vi "Data Processing.vi"(7 "Start Time Stamp":timestamp, 8 "error in":errorcluster, 9 "Control Data Notifier":refnum<notifier>, 10 "Unprocessed Data":refnum<queue>, 11 "Calibration Configuration":T2) -> (0 "error out":errorcluster, 2 "Data":T1, 3 "Data w Time":T1)   [LabVIEW 2024]
uses:
  support/Control/Waveform Data Constant.ctl
  Configuration/Calibration Configuration.ctl
  support/Control/Data Constant.ctl
  support/Control/Control Data Constant.ctl
  <vilib>/Analysis/baseanly.llb/Mean (DBL).vi
  <vilib>/Waveform/DTblOps.llb/DTbl Digital to Boolean Array.vi
  <vilib>/Analysis/NI_AALBase.lvlib
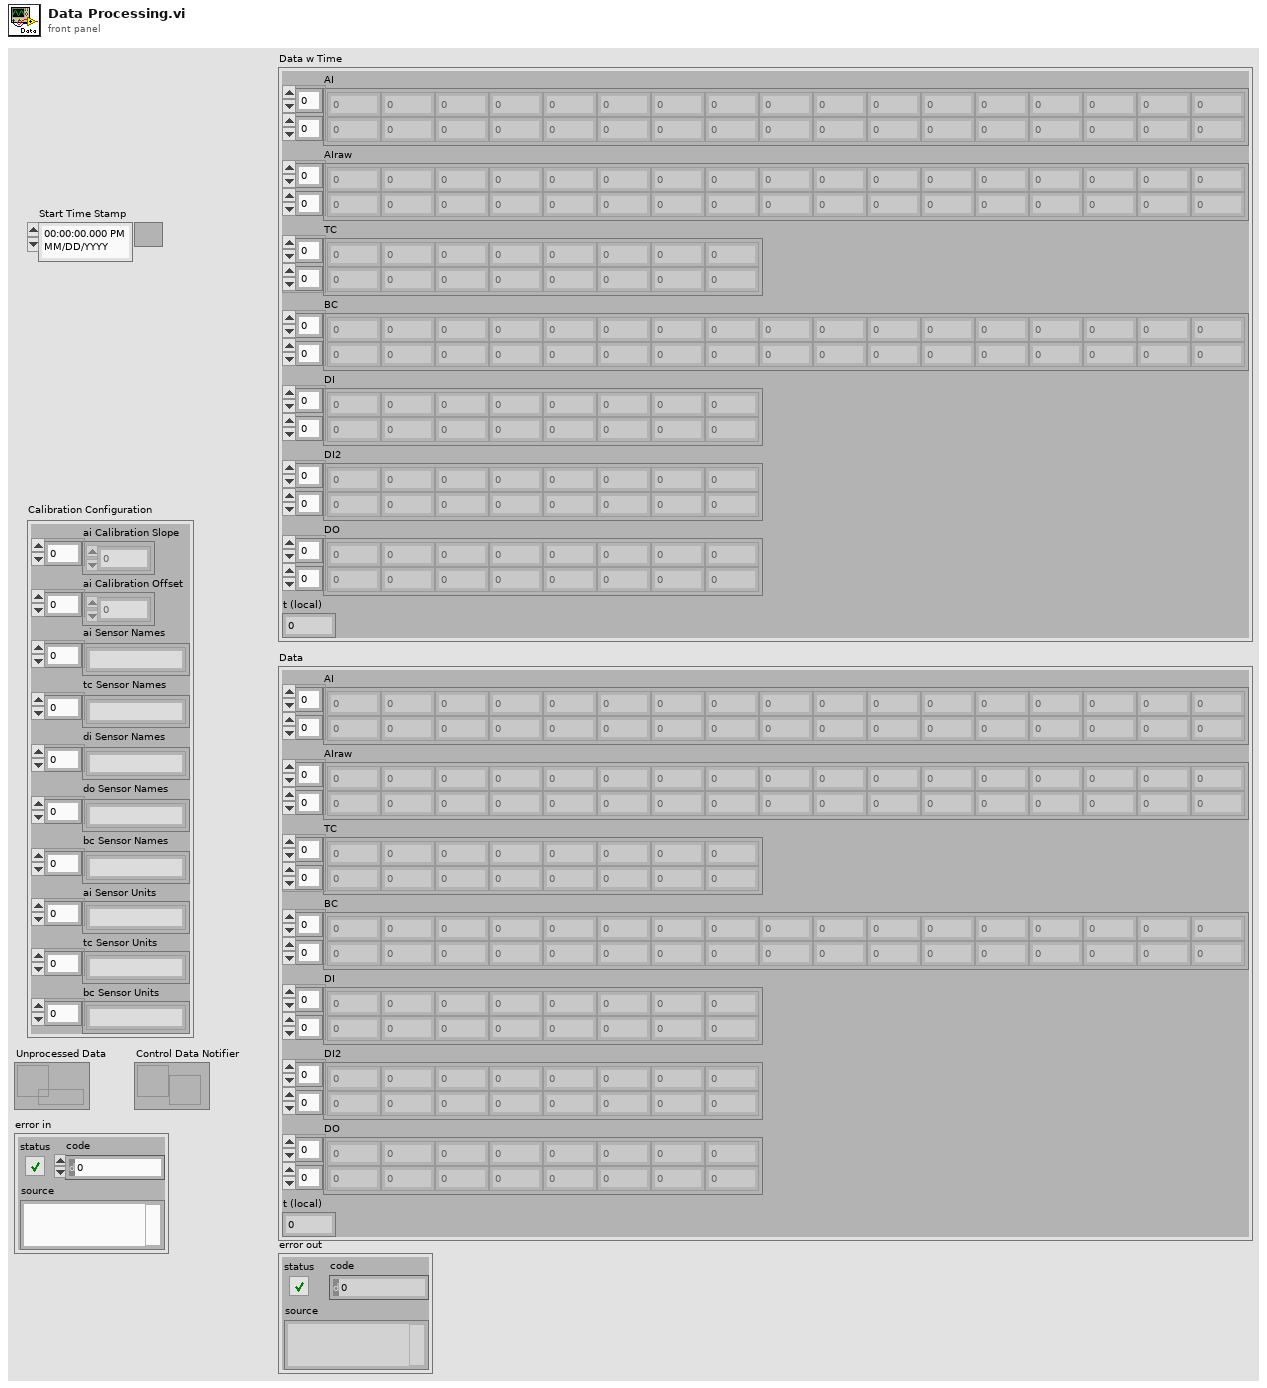
[diagram p1: front panel]
types:
  T1 = typedef "Data Constant.ctl" = cluster{"AI":dbl[][], "AIraw":dbl[][], "TC":dbl[][], "BC":dbl[][], "DI":dbl[][], "DI2":dbl[][], "DO":dbl[][], "t (local)":dbl}
  T2 = typedef "Calibration Configuration.ctl" = cluster{"ai Calibration Slope":dbl[], "ai Calibration Offset":dbl[], "ai Sensor Names ":string[], "tc Sensor Names":string[], "di Sensor Names":string[], "do Sensor Names":string[], "bc Sensor Names":string[], "ai Sensor Units":string[], "tc Sensor Units":string[], "bc Sensor Units":string[]}
  T3 = typedef "Waveform Data Constant.ctl" = cluster{"AI":waveform(dbl)[], "TC":waveform(dbl)[], "BC":waveform(dbl)[], "DI":digitalwaveform[], "DI2":digitalwaveform[]}
  T4 = typedef "Control Data Constant.ctl" = cluster{"Time (utc)":ext, "Data Out":cluster{"DO":bool[], "Module Number":string}[]}
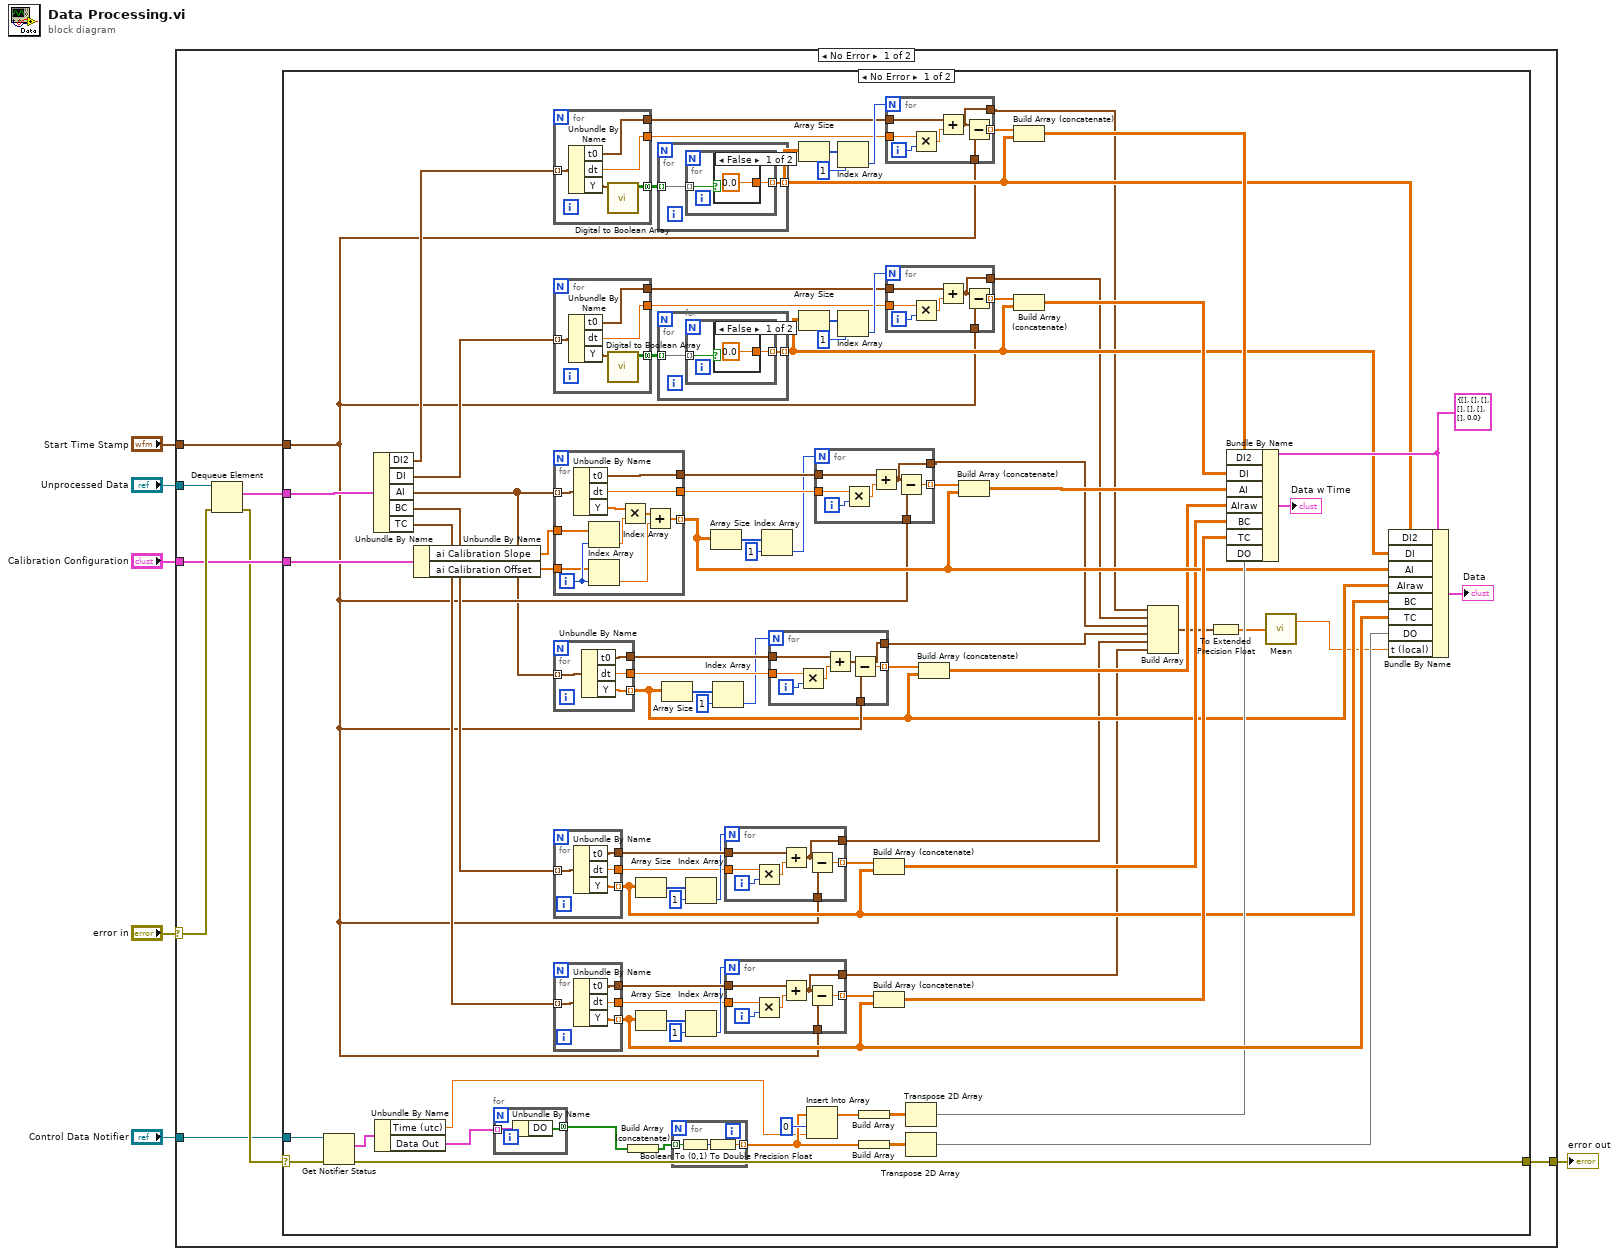
[diagram p0: block diagram]
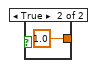
[diagram p2: hidden frame]
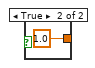
[diagram p3: hidden frame]
diagram:
  n1 = case shown="No Error" "error in" {
    selector: "error in" -> [w12 w194]
    tunnel: "Unprocessed Data" -> [w13 _]
    tunnel: [w9 w194] -> w4
    tunnel: "Calibration Configuration" -> [w11 _]
    tunnel: "Start Time Stamp" -> [w10 _]
    tunnel: "Control Data Notifier" -> [w7 _]
    frame No Error {
      n2 = Dequeue Element(queue=w13, error in (no error)=w12) -> (element=w14:T3, error out=w8:errorcluster)  [unwired: 1 in, 2 out]
      n3 = case shown="No Error" w8 {
        selector: w8 -> [w61 _]
        tunnel: w14 -> [w101 _]
        tunnel: w11 -> [w92 _]
        tunnel: w10 -> [w30 _]
        tunnel: [w60 _] -> w9
        tunnel: w7 -> [w64 _]
        frame No Error {
          w62 = T1 {"AI"=[], "AIraw"=[], "TC"=[], "BC"=[], "DI"=[], "DI2"=[], "DO"=[], "t (local)"=0.0} ("Data")
          n4 = Get Notifier Status(notifier=w64, error in (no error)=w61) -> (current notification=w42:T4, error out=w60:errorcluster)  [unwired: 3 out]
          n5 = Unbundle By Name(w101) -> ("DI2"=w52:digitalwaveform[], "DI"=w84:digitalwaveform[], "AI"=w29:waveform(dbl)[], "BC"=w80:waveform(dbl)[], "TC"=w95:waveform(dbl)[])
          n6 = Unbundle By Name(w42) -> ("Time (utc)"=w17:ext, "Data Out"=w16:cluster{"DO":bool[], "Module Number":string}[])
          n7 = Unbundle By Name(w92) -> ("ai Calibration Slope"=w91:dbl[], "ai Calibration Offset"=w90:dbl[])
          n8 = for {
            tunnel: w16 -> [w103] mode=indexing
            tunnel: [w102] -> w15 mode=concatenating
            n9 = Unbundle By Name(w103) -> ("DO"=w102:bool[])
          }
          n10 = for {
            tunnel: w52 -> [w128] mode=indexing
            tunnel: [w127] -> w55
            tunnel: [w126] -> w57 mode=concatenating
            tunnel: [w125] -> w54
            n11 = Unbundle By Name(w128) -> ("t0"=w127:timestamp, "dt"=w125:dbl, "Y"=w129:digitaldata)
            n12 = call-poly <vilib>:"Digital to Boolean Array.vi"("digital data"=w129) -> ("boolean array"=w126:bool[][])  [unwired: 9 in, 1 out]
          }
          n13 = for {
            tunnel: w84 -> [w164] mode=indexing
            tunnel: [w163] -> w67
            tunnel: [w162] -> w83 mode=concatenating
            tunnel: [w161] -> w66
            n14 = Unbundle By Name(w164) -> ("t0"=w163:timestamp, "dt"=w161:dbl, "Y"=w165:digitaldata)
            n15 = call-poly <vilib>:"Digital to Boolean Array.vi"("digital data"=w165) -> ("boolean array"=w162:bool[][])  [unwired: 9 in, 1 out]
          }
          n16 = for {
            tunnel: w29 -> [w193] mode=indexing
            tunnel: [w192] -> w97
            tunnel: [w191] -> w98
            tunnel: [w183] -> w39 mode=indexing
            tunnel: w91 -> [w185]
            tunnel: w90 -> [w184]
            i -> [w188]
            n17 = Unbundle By Name(w193) -> ("t0"=w192:timestamp, "dt"=w191:dbl, "Y"=w190:dbl[])
            n18 = Index Array(array=w185, index=w188) -> (element=w189:dbl)
            n19 = Index Array(array=w184, index=w188) -> (element=w186:dbl)
            n20 = Multiply(x=w190, y=w189) -> (x*y=w187:dbl[])
            n21 = Add(x=w187, y=w186) -> (x+y=w183:dbl[])
          }
          n22 = for {
            tunnel: w29 -> [w114] mode=indexing
            tunnel: [w113] -> w33
            tunnel: [w112] -> w34
            tunnel: [w111] -> w27 mode=indexing
            n23 = Unbundle By Name(w114) -> ("t0"=w113:timestamp, "dt"=w112:dbl, "Y"=w111:dbl[])
          }
          n24 = for {
            tunnel: w80 -> [w160] mode=indexing
            tunnel: [w159] -> w75
            tunnel: [w158] -> w73
            tunnel: [w157] -> w37 mode=indexing
            n25 = Unbundle By Name(w160) -> ("t0"=w159:timestamp, "dt"=w158:dbl, "Y"=w157:dbl[])
          }
          n26 = for {
            tunnel: w95 -> [w175] mode=indexing
            tunnel: [w174] -> w72
            tunnel: [w173] -> w70
            tunnel: [w172] -> w79 mode=indexing
            n27 = Unbundle By Name(w175) -> ("t0"=w174:timestamp, "dt"=w173:dbl, "Y"=w172:dbl[])
          }
          n28 = Build Array (concatenate)(w15) -> (w40:bool[])
          n29 = Array Size(array=w37) -> (size(s)=w81:i32[])
          n30 = Array Size(array=w79) -> (size(s)=w93:i32[])
          n31 = for {
            tunnel: w57 -> [w131] mode=indexing
            tunnel: [w130] -> w50 mode=indexing
            n32 = for {
              tunnel: w131 -> [w133] mode=indexing
              tunnel: [w132] -> w130 mode=indexing
              n33 = case shown="False" w133 {
                tunnel: [0.0 1.0] -> w132
                frame False {
                }
                frame True {
                }
              }
            }
          }
          n34 = for {
            tunnel: w83 -> [w167] mode=indexing
            tunnel: [w166] -> w41 mode=indexing
            n35 = for {
              tunnel: w167 -> [w169] mode=indexing
              tunnel: [w168] -> w166 mode=indexing
              n36 = case shown="False" w169 {
                tunnel: [0.0 1.0] -> w168
                frame False {
                }
                frame True {
                }
              }
            }
          }
          n37 = Array Size(array=w27) -> (size(s)=w35:i32[])
          n38 = for {
            tunnel: [w115] -> w43 mode=indexing
            tunnel: w40 -> [w117] mode=indexing
            n39 = Boolean To (0,1)(Boolean=w117) -> (0, 1=w116:i16)
            n40 = To Double Precision Float(number=w116) -> (double precision float=w115:dbl)
          }
          n41 = Index Array(array=w81, index=1) -> (element=w74:i32)
          n42 = Index Array(array=w93, index=1) -> (element=w71:i32)
          n43 = Array Size(array=w39) -> (size(s)=w99:i32[])
          n44 = Index Array(array=w35, index=1) -> (element=w31:i32)
          n45 = for {
            N: w74 -> [_]
            tunnel: w73 -> [w155]
            tunnel: w75 -> [w153]
            tunnel: [w152] -> w76 mode=indexing
            tunnel: w30 -> [w151]
            tunnel: [w150] -> w22
            i -> [w156]
            n46 = Multiply(x=w155, y=w156) -> (x*y=w154:dbl)
            n47 = Add(x=w153, y=w154) -> (x+y=w150:timestamp)
            n48 = Subtract(x=w150, y=w151) -> (x-y=w152:dbl)
          }
          n49 = for {
            N: w71 -> [_]
            tunnel: w70 -> [w148]
            tunnel: w72 -> [w146]
            tunnel: [w145] -> w69 mode=indexing
            tunnel: w30 -> [w144]
            tunnel: [w143] -> w19
            i -> [w149]
            n50 = Multiply(x=w148, y=w149) -> (x*y=w147:dbl)
            n51 = Add(x=w146, y=w147) -> (x+y=w143:timestamp)
            n52 = Subtract(x=w143, y=w144) -> (x-y=w145:dbl)
          }
          n53 = Index Array(array=w99, index=1) -> (element=w89:i32)
          n54 = for {
            N: w31 -> [_]
            tunnel: w34 -> [w109]
            tunnel: w33 -> [w107]
            tunnel: [w106] -> w32 mode=indexing
            tunnel: w30 -> [w105]
            tunnel: [w104] -> w23
            i -> [w110]
            n55 = Multiply(x=w109, y=w110) -> (x*y=w108:dbl)
            n56 = Add(x=w107, y=w108) -> (x+y=w104:timestamp)
            n57 = Subtract(x=w104, y=w105) -> (x-y=w106:dbl)
          }
          n58 = Array Size(array=w50) -> (size(s)=w59:i32[])
          n59 = Array Size(array=w41) -> (size(s)=w86:i32[])
          n60 = Insert Into Array(array=w43, index=0, new element=w17) -> (w49:dbl[])
          n61 = for {
            N: w89 -> [_]
            tunnel: w98 -> [w181]
            tunnel: w97 -> [w179]
            tunnel: [w178] -> w96 mode=indexing
            tunnel: w30 -> [w177]
            tunnel: [w176] -> w24
            i -> [w182]
            n62 = Multiply(x=w181, y=w182) -> (x*y=w180:dbl)
            n63 = Add(x=w179, y=w180) -> (x+y=w176:timestamp)
            n64 = Subtract(x=w176, y=w177) -> (x-y=w178:dbl)
          }
          n65 = Index Array(array=w59, index=1) -> (element=w56:i32)
          n66 = Index Array(array=w86, index=1) -> (element=w68:i32)
          n67 = Build Array(w49) -> (w47:dbl[][])
          n68 = Build Array(w43) -> (w46:dbl[][])
          n69 = Build Array (concatenate)(w76, w37) -> (w38:dbl[][])
          n70 = Build Array (concatenate)(w69, w79) -> (w78:dbl[][])
          n71 = for {
            N: w56 -> [_]
            tunnel: w54 -> [w123]
            tunnel: w55 -> [w121]
            tunnel: [w120] -> w53 mode=indexing
            tunnel: w30 -> [w119]
            tunnel: [w118] -> w26
            i -> [w124]
            n72 = Multiply(x=w123, y=w124) -> (x*y=w122:dbl)
            n73 = Add(x=w121, y=w122) -> (x+y=w118:timestamp)
            n74 = Subtract(x=w118, y=w119) -> (x-y=w120:dbl)
          }
          n75 = for {
            N: w68 -> [_]
            tunnel: w66 -> [w141]
            tunnel: w67 -> [w139]
            tunnel: [w138] -> w65 mode=indexing
            tunnel: w30 -> [w137]
            tunnel: [w136] -> w25
            i -> [w142]
            n76 = Multiply(x=w141, y=w142) -> (x*y=w140:dbl)
            n77 = Add(x=w139, y=w140) -> (x+y=w136:timestamp)
            n78 = Subtract(x=w136, y=w137) -> (x-y=w138:dbl)
          }
          n79 = Transpose 2D Array(2D array=w47) -> (transposed array=w45:dbl[][])
          n80 = Transpose 2D Array(2D array=w46) -> (transposed array=w44:dbl[][])
          n81 = Build Array (concatenate)(w32, w27) -> (w28:dbl[][])
          n82 = Build Array (concatenate)(w96, w39) -> (w87:dbl[][])
          n83 = Build Array (concatenate)(w53, w50) -> (w51:dbl[][])
          n84 = Build Array (concatenate)(w65, w41) -> (w88:dbl[][])
          n85 = Build Array(w26, w25, w24, w23, w22, w19) -> (w21:timestamp[])
          n86 = To Extended Precision Float(1:w21) -> (0:w20:ext[])
          n87 = Bundle By Name(cluster=w62, "DI2"=w51, "DI"=w88, "AI"=w87, "AIraw"=w28, "BC"=w38, "TC"=w78, "DO"=w45) -> (→"Data w Time":T1)
          n88 = call-poly <vilib>:"Mean.vi"("X"=w20) -> ("mean"=w18:dbl)  [unwired: 1 out]
          n89 = Bundle By Name(cluster=w62, "DI2"=w50, "DI"=w41, "AI"=w39, "AIraw"=w27, "BC"=w37, "TC"=w79, "DO"=w44, "t (local)"=w18) -> (→"Data":T1)
        }
        frame Error {
        }
      }
    }
    frame Error {
    }
  }
  "error out" <- w4
